vi "Parse Str Ctl and Variant.vi"(8 "error in":errorcluster, 11 "String Input":string) -> (0 "error out":errorcluster, 2 "variant output":variant, 3 "Control Name":string)   [LabVIEW 2020]
doc: "Parses an ended string to extract the prepended control name, the array of types and the variant data.\n\n(c) 2022 Scott Hannahs <sth@magnet.fsu.edu>\nVersion 1 9/23/2022"
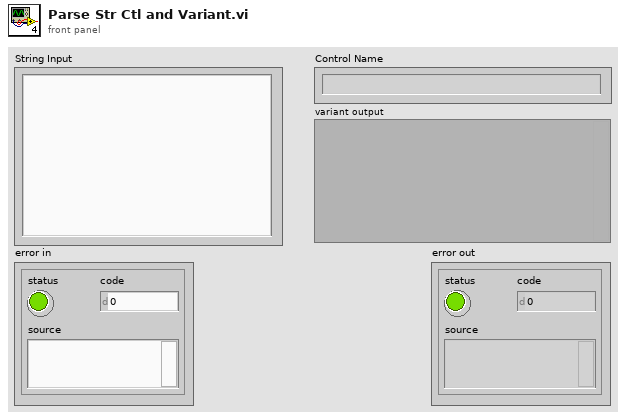
[diagram p1: front panel]
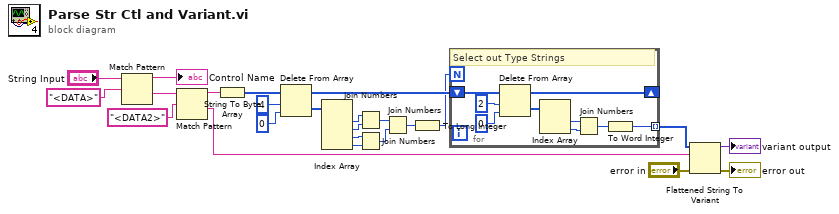
[diagram p0: block diagram]
diagram:
  n1 = Match Pattern(string="String Input", regular expression="<DATA>") -> (before substring=→"Control Name":string, after substring=w9:string)  [unwired: 1 in, 2 out]
  n2 = Match Pattern(string=w9, regular expression="<DATA2>") -> (before substring=w8:string, after substring=w6:string)  [unwired: 1 in, 2 out]
  n3 = String To Byte Array(string=w8) -> (unsigned byte array=w14:u8[])
  n4 = Delete From Array(array=w14, length=4, index=0) -> (deleted portion=w13:u8[], array with subset deleted=w12:u8[])
  n5 = Index Array(array=w13) -> (element #1=w23:u8, element #2=w22:u8, element #3=w21:u8, element #4=w20:u8)  [unwired: 4 in]
  n6 = Join Numbers(hi=w23, lo=w22) -> ((hi.lo)=w18:u16)
  n7 = Join Numbers(hi=w21, lo=w20) -> ((hi.lo)=w19:u16)
  n8 = Join Numbers(hi=w18, lo=w19) -> ((hi.lo)=w17:u32)
  n9 = To Long Integer(number=w17) -> (32bit integer=w3:i32)
  n10 = for {
    N: w3 -> [_]
    shift-right: [w32] -> _
    shift-left: w12 -> [w33]
    tunnel: [w25] -> w7 mode=indexing
    # "Select out Type Strings"
    n11 = Delete From Array(array=w33, length=2, index=0) -> (deleted portion=w30:u8[], array with subset deleted=w32:u8[])
    n12 = Index Array(array=w30) -> (element #1=w29:u8, element #2=w28:u8)  [unwired: 2 in]
    n13 = Join Numbers(hi=w29, lo=w28) -> ((hi.lo)=w27:u16)
    n14 = To Word Integer(number=w27) -> (16bit integer=w25:i16)
  }
  n15 = Flattened String To Variant(4:"error in", 6:w6, 7:w7) -> (0:→"error out":errorcluster, 3:→"variant output":variant)
